vi "Module Init.vi"(8 "error in (no error)":errorcluster, 11 "Log Preparer Module in":refnum<class "Log Preparer Module.lvclass">) -> (0 "error out":errorcluster, 3 "Log Preparer Module out":refnum<class "Log Preparer Module.lvclass">)   [LabVIEW 2020, in "VolatusData.lvlib" / "Log Preparer Module.lvclass"]
uses:
  Log Preparer Module.lvclass
  C:/dev/lv20CE/relink/lv-volatus/Volatus/Module/Module.lvclass
  Volatus/Module/Module.lvclass/Module.ctl
  Volatus/MessageQ/MessageQ.lvclass/MessageQ.ctl
  Volatus/Module/Self Q.vi
  Volatus/MessageQ/Send.vi
  Volatus/Module/Module.lvclass
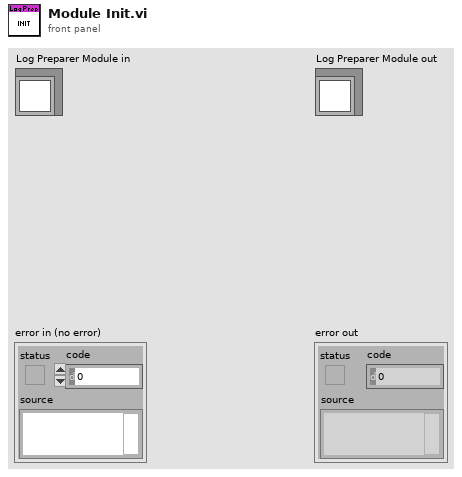
[diagram p1: front panel]
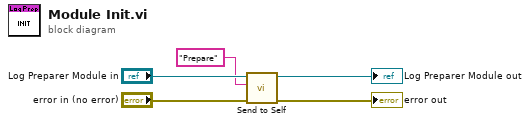
[diagram p0: block diagram]
diagram:
  n1 = call "Send to Self.vi"("error in (no error)"="error in (no error)", "Message ID"="Prepare", "Module in"="Log Preparer Module in") -> ("error out"=→"error out":errorcluster, "Module out"=→"Log Preparer Module out":refnum<class "Log Preparer Module.lvclass">)  [unwired: 7 in]
